vi "Byte_buffer_flush.vi"(11 "reference":refnum<visa-resource-name>) -> ()   [LabVIEW 2017]
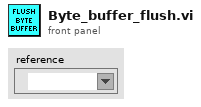
[diagram p1: front panel]
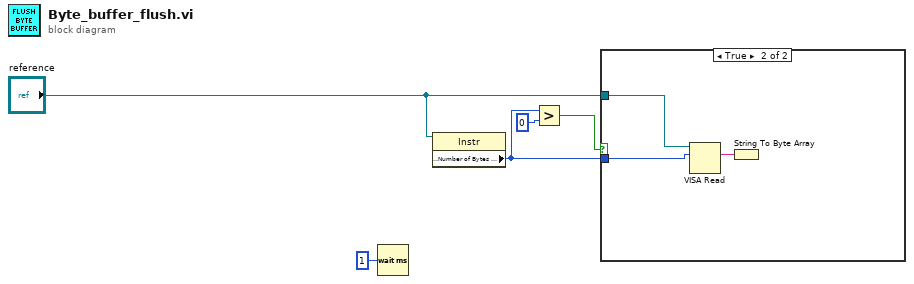
[diagram p0: block diagram]
diagram:
  n1 = Wait (ms)(milliseconds to wait=u32 1) -> ()  [unwired: 1 out]
  n2 = property class="Instr"(reference="reference") -> ("Serial Settings:Number of Bytes at Serial Port"=w4:u32)  [unwired: 1 in, 2 out]
  n3 = Greater?(x=w4, y=u32 0) -> (0:w1:bool)
  n4 = case shown="True" w1 {
    tunnel: w4 -> [_ w8]
    tunnel: "reference" -> [_ w7]
    frame False {
    }
    frame True {
      n5 = VISA Read(VISA resource name=w7, byte count=w8) -> (read buffer=w6:string)  [unwired: 1 in, 3 out]
      n6 = String To Byte Array(string=w6) -> ()  [unwired: 1 out]
    }
  }
